vi "Value Entry_DBL.vi"(11 "Value In":dbl) -> (2 "Apply":bool, 3 "Value Out":dbl)   [LabVIEW 2018, in "Tag Watchlist.lvlib"]
uses:
  Tag Watchlist.lvlib
panel:
  in  "Cancel":bool
  in  "OK":bool
  in  "Value":dbl caption="New Value"
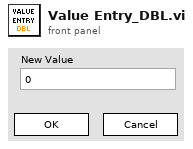
[diagram p1: front panel]
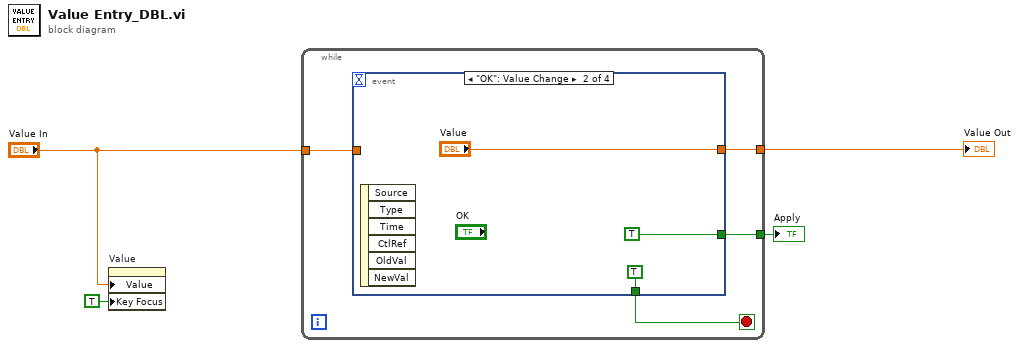
[diagram p0: block diagram]
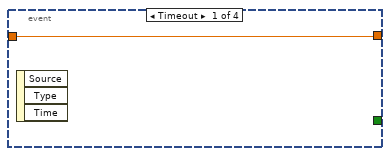
[diagram p2: hidden frame]
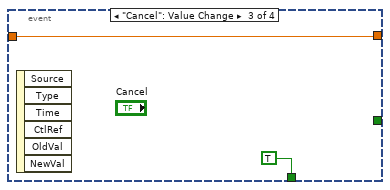
[diagram p3: hidden frame]
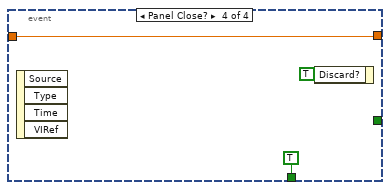
[diagram p4: hidden frame]
diagram:
  n1 = property on="Value" class="DigNum (strict)"("Value"="Value In", "Key Focus"=TRUE) -> ()  [unwired: 2 in, 2 out]
  n2 = while {
    tunnel: "Value In" -> [w8]
    tunnel: [w7] -> w4
    tunnel: [w5] -> w3
    stop <- w6 stop-if-true
    n3 = event shown="[1] \"OK\": Value Change" {
      selector: _ -> [_ _ _ _]
      dyn-events: _ -> [_ _ _ _]
      timeout: _ -> [_ _ _ _]
      tunnel: w8 -> [w9 _ w13 w15]
      tunnel: [w9 "Value" w13 w15] -> w7
      tunnel: [_ TRUE TRUE TRUE] -> w6
      tunnel: [_ TRUE _ _] -> w5
      event Timeout {
        n4 = event-data() -> ()  [unwired: 1 in, 3 out]
      }
      event "OK": Value Change {
        n5 = event-data() -> ()  [unwired: 1 in, 6 out]
      }
      event "Cancel": Value Change {
        n6 = event-data() -> ()  [unwired: 1 in, 6 out]
      }
      event Panel Close? {
        n7 = event-data() -> ()  [unwired: 1 in, 4 out]
        n8 = event-data("Discard?"=TRUE) -> ()  [unwired: 1 in, 1 out]
      }
    }
  }
  "Value Out" <- w4
  "Apply" <- w3
